vi "ACP_Display.vi"(7 "ACP_Values":dbl[](array[numeric]) format="%#_6p", 8 "Int_Bandwidth":dbl[](array[numeric]) format="%#_6p", 9 "Offsets":dbl[](array[numeric]) format="%#_6p", 10 "SignalBandwidth":dbl format="%#_6p", 11 "Input_Waveform":cluster{"t0":dbl, "dt":dbl, "Y":dbl[]}={"t0"=984962406.0150375, "dt"=75187.96992481203, "Y"=[-89.63999973694473, -88.64929239598041, -87.72298465887505, -87.8672826941664, -89.71738802076464, -91.38617840455802, -89.85619847441421, -88.23187719443631, -88.31178816897933, -90.00303942484523, -91.8121579546794, -90.6131823061693, -88.6020694172166, -87.37396848650413, -86.59799080201411, -86.18839913393768, -86.42502772343161, -87.7982557697421, -90.02492665073716, -90.4415866092301, -88.92788112009788, -88.29826990448431, -87.39483113612397, -85.7998254046862, -85.63115765746092, -86.95627476729193, -87.2640795687788, -86.24568886575666, -85.50151482449424, -85.51002261382666, -86.37279849031779, -88.01238210307704, -89.43301513785883, -88.92673622763284, -88.4348792730645, -89.21935963997967, -89.46134971051514, -88.99542983202693, -88.27463910135603, -88.13774805838604, -89.19562416795786, -89.92705558861087, -90.09082163589055, -88.69362278061517, -87.31616795736572, -87.11386448675165, -87.23068106767897, -86.67936200942775, -86.49215985938753, -87.51370123772816, -88.06251133265317, -86.69110401881747, -85.29690704193632, -84.6960839018393, -84.79019374286301, -84.885793540852, -84.63311974169622, -84.55712193577551, -85.1041619251538, -85.91493120502224, -86.982301367372, -88.0832306079449, -87.8510306637505, -86.67536532865142, -86.12713810151233, -86.35364342835851, -87.21263973263733, -88.05046484514821, -88.25762691873729, -88.43415782442676, -87.55557794001312, -86.60044078952595, -86.23322411161615, -85.47129715526728, -85.72780720644495, -87.06917230159392, -86.03428667048773, -84.10315597541745, -83.61540573293807, -84.69525157791979, -86.45046234162324, -85.63735590514283, -84.46067124295938, -85.00452353107816, -85.59321976179615, -85.20307931282638, -85.31559620968477, -86.30273561160791, -85.7108125814753, -84.88195194194469, -87.26693415560972, -89.40843802100842, -86.8072131726059, -85.98560167091048, -86.02257122479479, -85.02800086804983, -84.01433583431013, -83.95967580538382, -84.63208081876799, -85.48745909079923, -85.45691946012826, -84.55308992211484, -84.16269530732643, -85.43763643600357, -87.11386260132592, -87.23982610686313, -87.71190675663709, -88.28216301960768, -87.59930592585448, -86.5883557989581, -85.71558795807199, -84.15017709878046, -82.38610626891705, -81.97124915901372, -83.28830849833354, -84.98885235666548, -84.96164572749652, -85.5843473244137, -88.56252490920488, -87.64620036056482, -84.96475660703327, -85.55109208743959, -86.83523831530445, -85.536663502489, -85.44885323517255, -87.68790672782528, -88.75971118611534, -87.67564577265638, -88.54109466243108, -85.29800873432679, -74.4898463968675, -63.0326443950114, -55.17922511945281, -51.33220943316353, -51.453959961321104, -55.589554860594546, -64.61456694978114, -67.4812778941181, -48.489809932679265, -35.802240925096356, -26.730177710528224, -20.735711602154716, -17.2982390365364, -16.030102222531873, -16.835839734133764, -19.839126374391924, -25.319870860768432, -35.86639924634176, -38.79850444284489, -31.24244407213132, -25.87842731534778, -21.25804549078628, -19.290297059713176, -21.378078990032257, -27.305789901115062, -20.59604245481927, -18.72094002613551, -22.840057971500904, -35.761629640346385, -42.155364948558116, -23.958556681249924, -18.3741929613444, -17.163055494253655, -18.407742033316495, -21.84958526019429, -24.35320534201672, -19.4901058881642, -16.13706137982578, -15.2985080678029, -16.834891831867992, -21.14088210837319, -24.27136962775262, -21.347229401507086, -21.98712998415924, -31.37973461481362, -25.223360423680205, -18.535631332230963, -16.91735061328471, -17.86668959656393, -20.688792379578885, -22.375011000775977, -21.017138743137743, -21.33034377305904, -23.631513483150727, -25.99083690044359, -28.472051240197914, -32.293943871014605, -27.54753306684772, -21.03112670687183, -17.995389637069586, -17.96375064029052, -19.77653238577541, -21.213226874941917, -22.96821139654955, -28.347585293349667, -23.986529989110295, -18.29983136493145, -15.694060632891407, -14.632591706040934, -14.972856500342829, -16.855226002405892, -20.353589515147718, -25.512679846354544, -29.254474871912812, -29.834413252676136, -24.317430059466155, -20.265782179316993, -20.770358765304834, -24.80623413878626, -21.395369020392906, -20.525767415261562, -22.52914946160388, -24.48832478758139, -24.985875038373187, -23.39727894109801, -30.6436234950965, -29.00717047333317, -29.866044960605862, -22.024856306867107, -17.568589490591506, -18.830051410700563, -21.117132967879073, -21.095107620512287, -19.74972621750463, -17.009629441659662, -15.654366671424931, -16.295789864325457, -19.89392747707796, -30.668156349931152, -33.146059945221964, -23.73426792975797, -18.206127995199097, -15.51488774168675, -14.691984312156166, -15.324946839685346, -17.705313343094026, -22.139540379286636, -26.87854482392156, -25.98135289765947, -23.39789846232484, -25.022358323136537, -36.83605879101415, -25.856961385975907, -20.721404533919305, -19.184464703333077, -20.641755732846818, -23.134446196330373, -24.591277401941795, -29.58362395392095, -26.0000745073865, -18.68585403337235, -16.003898645922263, -15.363760634785734, -15.20503122873891, -15.910613257458266, -17.020268273866208, -16.417384785082305, -14.333984084628568, -13.314083201127346, -14.727413327441312, -19.10167293251652, -26.764939572466197, -38.09155891460742, -53.64279033876912, -69.36288059848718, -65.75502798430428, -60.96903389437804, -60.3938137236956, -63.90683277709688, -71.03691234836879, -78.69263934382148, -82.09262129299444, -83.18584750454336, -83.82037606561262, -83.80436899397816, -83.46060159419221, -84.877485269554, -87.93160459313725, -88.1421354425784, -87.13140155563217, -84.70219514509957, -83.05738790157994, -83.26207706474035, -84.29430296548927, -83.79435656720675, -81.58868601062619, -80.26788357608308, -80.26523793285749, -80.76317879510272, -81.61141184216635, -83.17032559509107, -84.33177236541441, -83.3129112639014, -82.56736385330164, -83.6335003542586, -85.70618433084329, -86.8162509259204, -87.0635648611678, -87.32299422763194, -86.99798796564524, -86.41361664780422, -86.36127964474366, -87.04348720411012, -87.71940041627147, -86.4223418894893, -85.0948235390574, -85.30989108065572, -87.10893161289705, -87.18169079994395, -83.91001776034172, -82.10465576810678, -82.43603882084842, -83.99752955540932, -84.59011781015084, -83.68043201240793, -82.7167093523576, -82.9961245480711, -85.29964052285244, -88.51979429386886, -88.18892949097733, -86.24526836345623, -85.26096599458748, -85.22853297873162, -86.45140265843743, -89.2818438656248, -92.55038126432652, -91.27626274119564, -88.21324776476074, -86.52540906046747, -86.2233392829663, -85.70997679843697, -84.86798358161464, -85.46194686598113, -87.58326634176515, -88.4783548469245, -88.02838629290386, -88.30735250313893, -88.10163547548203, -86.52569182875922, -85.3686642703778, -85.55251311930887, -86.06649726533341, -86.66630194425761, -87.89214928230007, -88.64884148075299, -87.23109120058412, -85.61583947996715, -85.37067361550072, -86.93725820486779, -89.6886025379761, -90.10798115629774, -89.4084073952703, -89.03163163344618, -89.34179336433778, -89.28789884507763, -87.9106340163687, -86.59687158814671, -85.3338484400389, -84.36603857205044, -84.20103140119174, -85.22167579722877, -87.49154452532767, -89.51815520852844, -88.57204532824198, -87.05390275033501, -86.2104833613782, -86.00550423669743, -86.0362616714008, -85.72290852913369, -84.79385962022485, -84.18592858987722, -85.2315507413144, -87.7903275512613, -88.8687941922862, -87.93256878083358, -87.27118803570661, -87.47863599510785, -88.50521728218285, -88.80472315769815, -88.56376328887107, -89.15596226313185, -89.1517085064617, -89.04183876937535, -88.91994300682859, -89.08042438597633, -89.88258945023176, -90.32661076475101, -91.32635361976908, -91.03754531406253, -88.55664943821515, -86.93548005757741, -86.75251731440254, -88.3168249079199, -91.13744800816669, -92.3599441562213, -91.250837470247, -90.50215071133562, -90.58083600186505, -90.42183237810697, -89.63999973694473]}) -> (3 "Waveform Graph 2":cluster{"t0":dbl, "dt":dbl, "Y":dbl[]}[](graph))   [LabVIEW 2014]
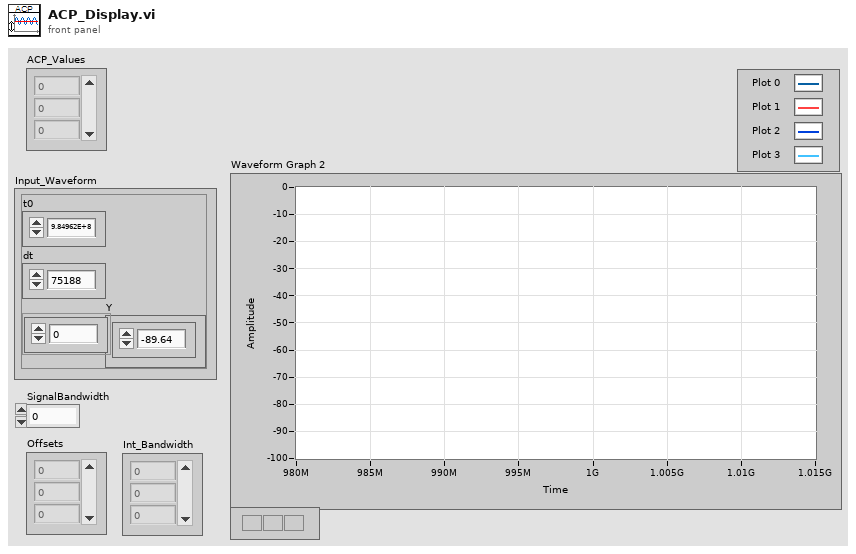
[diagram p1: front panel]
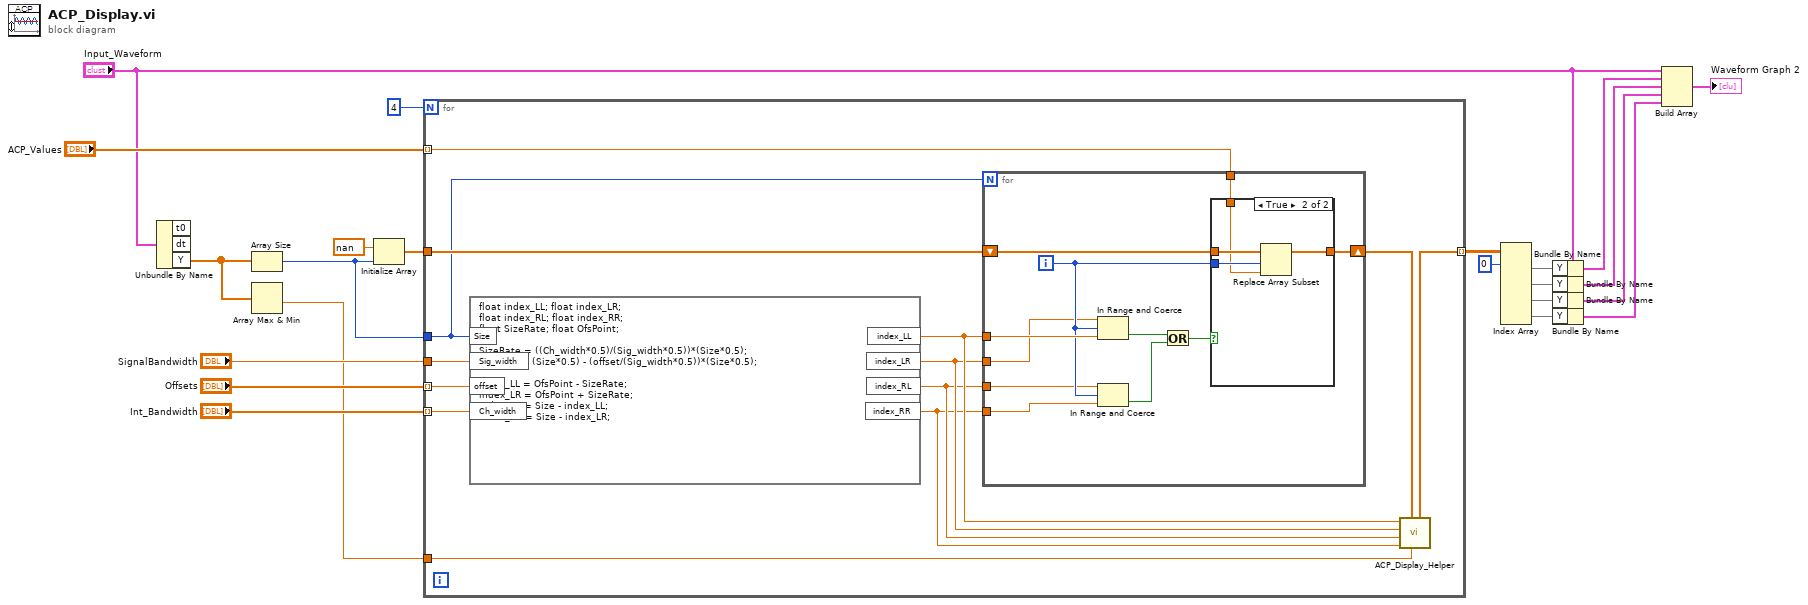
[diagram p0: block diagram]
diagram:
  n1 = Unbundle By Name("Input_Waveform") -> ("Y"=w8:dbl[])  [unwired: 2 out]
  n2 = Array Size(array=w8) -> (size(s)=w6:i32)
  n3 = Array Max & Min(array=w8) -> (min value=w1:dbl)  [unwired: 3 out]
  n4 = Initialize Array(nan ("element"), w6) -> (w7:dbl[])
  n5 = for {
    N: 4 -> [_]
    tunnel: "SignalBandwidth" -> [w35]
    tunnel: "Offsets" -> [w34] mode=indexing
    tunnel: "Int_Bandwidth" -> [w33] mode=indexing
    tunnel: [w29] -> w17 mode=indexing
    tunnel: w7 -> [w31]
    tunnel: "ACP_Values" -> [w32] mode=indexing
    tunnel: w6 -> [w30]
    tunnel: w1 -> [w23]
    n6 = formula code="float index_LL; float index_LR;\nfloat index_RL; float index_RR; \nfloat SizeRate; float OfsPoint;\n\nSizeRate = ((Ch_width*0.5)/(Sig_width*0.5))*(Size*0.5);\nOfsPoint = (Size*0.5) - (offset/(Sig_width*0.5))*(Size*0.5);\n\nindex_LL = OfsPoint - SizeRate;\nindex_LR = OfsPoint + SizeRate;\nindex_RL = Size - index_LL;\nindex_RR = Size - index_LR;"("Sig_width"=w35, "offset"=w34, "Ch_width"=w33, "Size"=w30) -> ("index_LL"=w27:dbl, "index_LR"=w26:dbl, "index_RL"=w25:dbl, "index_RR"=w24:dbl)
    n7 = for {
      N: w30 -> [_]
      shift-right: [w44] -> w28
      shift-left: w31 -> [w45]
      tunnel: w27 -> [w46]
      tunnel: w25 -> [w38]
      tunnel: w24 -> [w39]
      tunnel: w26 -> [w37]
      tunnel: w32 -> [w36]
      i -> [w40]
      n8 = In Range and Coerce(upper limit=w37, x=w40, lower limit=w46) -> (In Range?=w43:bool)  [unwired: 1 out]
      n9 = In Range and Coerce(upper limit=w38, x=w40, lower limit=w39) -> (In Range?=w41:bool)  [unwired: 1 out]
      n10 = Or(x=w43, y=w41) -> (x .or. y?=w42:bool)
      n11 = case shown="True" w42 {
        tunnel: w45 -> [w47 w51]
        tunnel: w40 -> [_ w50]
        tunnel: [w47 w49] -> w44
        tunnel: w36 -> [_ w48]
        frame False {
        }
        frame True {
          n12 = Replace Array Subset(array=w51, new element=w48, index=w50) -> (w49:dbl[])
        }
      }
    }
    n13 = call "ACP_Display_Helper.vi"("Min"=w23, "Mask"=w28, "RR"=w24, "RL"=w25, "LR"=w26, "LL"=w27) -> ("Mask_Out"=w29:dbl[])  [unwired: 5 in]
  }
  n14 = Index Array(array=w17, index (row) #1=0 ("index (row)")) -> (element #1=w14:dbl[], element #2=w13:dbl[], element #3=w12:dbl[], element #4=w4:dbl[])  [unwired: 7 in]
  n15 = Bundle By Name(cluster="Input_Waveform", "Y"=w14) -> (w15:cluster{"t0":dbl, "dt":dbl, "Y":dbl[]})
  n16 = Bundle By Name(cluster="Input_Waveform", "Y"=w13) -> (w11:cluster{"t0":dbl, "dt":dbl, "Y":dbl[]})
  n17 = Bundle By Name(cluster="Input_Waveform", "Y"=w12) -> (w10:cluster{"t0":dbl, "dt":dbl, "Y":dbl[]})
  n18 = Bundle By Name(cluster="Input_Waveform", "Y"=w4) -> (w3:cluster{"t0":dbl, "dt":dbl, "Y":dbl[]})
  n19 = Build Array("Input_Waveform", w15, w11, w10, w3) -> (→"Waveform Graph 2":cluster{"t0":dbl, "dt":dbl, "Y":dbl[]}[])
